vi "Write enable C.vi"(8 "error in (no error)":errorcluster, 10 "enable C":bool, 11 "Trigger in":refnum<class "Trigger.lvclass">) -> (0 "error out":errorcluster, 3 "Trigger out":refnum<class "Trigger.lvclass">)   [LabVIEW 2018, in "Trigger.lvclass"]
uses:
  Trigger.lvclass
  Trigger.lvclass/Trigger.ctl
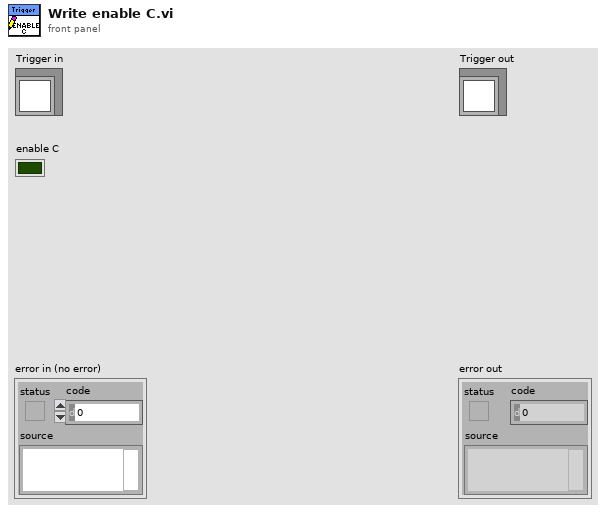
[diagram p1: front panel]
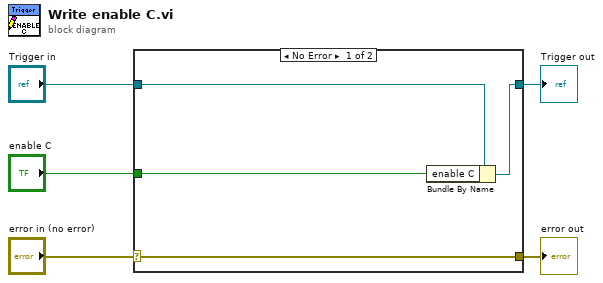
[diagram p0: block diagram]
diagram:
  n1 = case shown="No Error" "error in (no error)" {
    selector: "error in (no error)" -> [w9 w10]
    tunnel: [w9 w10] -> w4
    tunnel: [w7 w11] -> w2
    tunnel: "Trigger in" -> [w8 w11]
    tunnel: "enable C" -> [w6 _]
    frame No Error {
      n2 = Bundle By Name(cluster=w8, "enable C"=w6) -> (w7:refnum<class "Trigger.lvclass">)
    }
    frame Error {
    }
  }
  "error out" <- w4
  "Trigger out" <- w2
